vi "RelayControl.vi"(7 "Neutron Shutter":bool, 8 "Error In":errorcluster, 9 "Sample Space Pump":bool, 10 "Siphon Pump":bool, 11 "Relay In":refnum<visa-resource-name>) -> (0 "Error Out":errorcluster, 3 "Relay Out":refnum<visa-resource-name>)   [LabVIEW 2018]
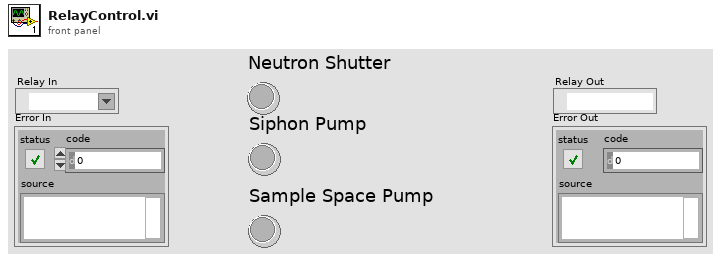
[diagram p1: front panel]
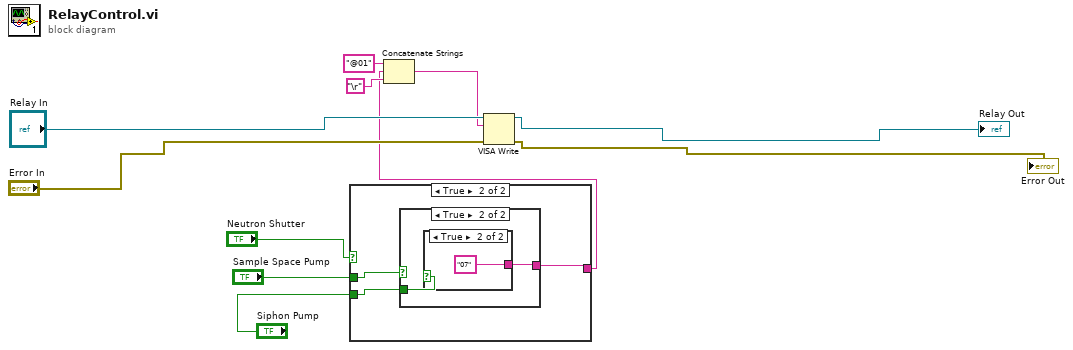
[diagram p0: block diagram]
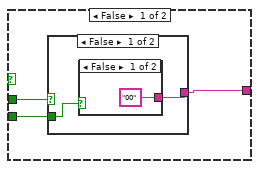
[diagram p2: hidden frame]
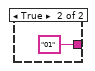
[diagram p3: hidden frame]
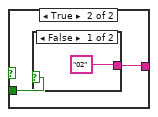
[diagram p4: hidden frame]
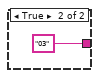
[diagram p5: hidden frame]
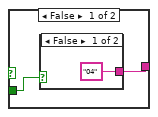
[diagram p6: hidden frame]
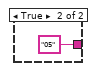
[diagram p7: hidden frame]
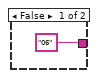
[diagram p8: hidden frame]
diagram:
  n1 = case shown="True" "Neutron Shutter" {
    tunnel: "Sample Space Pump" -> [w14 w24]
    tunnel: "Siphon Pump" -> [w13 w25]
    tunnel: [w12 w23] -> w2
    frame False {
      n2 = case shown="False" w14 {
        tunnel: w13 -> [w16 w20]
        tunnel: [w15 w19] -> w12
        frame False {
          n3 = case shown="False" w16 {
            tunnel: ["00" "01"] -> w15
            frame False {
            }
            frame True {
            }
          }
        }
        frame True {
          n4 = case shown="False" w20 {
            tunnel: ["02" "03"] -> w19
            frame False {
            }
            frame True {
            }
          }
        }
      }
    }
    frame True {
      n5 = case shown="True" w24 {
        tunnel: w25 -> [w27 w31]
        tunnel: [w26 w30] -> w23
        frame False {
          n6 = case shown="False" w27 {
            tunnel: ["04" "05"] -> w26
            frame False {
            }
            frame True {
            }
          }
        }
        frame True {
          n7 = case shown="True" w31 {
            tunnel: ["06" "07"] -> w30
            frame False {
            }
            frame True {
            }
          }
        }
      }
    }
  }
  n8 = Concatenate Strings("@01" ("string"), w2, "\r") -> (w5:string)
  n9 = VISA Write(VISA resource name="Relay In", write buffer=w5, error in (no error)="Error In") -> (VISA resource name out=→"Relay Out":refnum<visa-resource-name>, error out=→"Error Out":errorcluster)  [unwired: 1 out]
